vi "field emission sensor_v72.vi"() -> ()   [LabVIEW 2014]
uses:
  Keithley 24XX/Public/Data/Read (Single Point).vi
  Keithley 24XX/Keithley 24XX.lvlib
  <userlib>/Nanonis Prog Interface V5/Nanonis Prog Interface.lvlib
  <vilib>/Analysis/NI_AALBase.lvlib
panel:
  in  "p Current Amplitude (A)":dbl=-0.3 format="%#_6p"
  in  "Current Amplitude Max (A)":sgl=1.5e-10 format="%#_6p"
  in  "Std threshold":dbl=5e-12 format="%#_6p"
  in  "Mean threshold":dbl=2e-11 format="%#_6p"
  out "ramp paused":bool
  out "x+y":sgl=1.4799449e-10
  out "amplitude":sgl(graph)=1.0739469e-11
  in  "Amplitude (V) (NaN=no change)":sgl=nan
  in  "Frequency (Hz) (NaN=no change)":sgl=nan format="%#_6p"
  in  "p Amplitude":dbl=-0.3 format="%#_6p"
  in  "amplitude max":sgl=1.5e-10 format="%#_6p"
  in  "Signal index (0-79)":i8=49
  out "amplitude":sgl=1.0739469e-11 format="%#_6p"
  in  "dz":dbl=1e-09 format="%#_6p"
  in  "ramp delay (s)":dbl=0.001
  out "ramp trigger":bool
  out "millisecond timer value":u32=272952714
  in  "Clear plots":bool
  out "z":dbl(graph)=7.783200430924225e-08
  in  "Ramp":bool
  in  "steps":sgl=5e-09 format="%#_6p"
  in  "Ramp to":sgl=1.3e-06 format="%#_6p"
  in  "I":sgl=5e-05 format="%#_6p"
  in  "PID":bool
  in  "p":sgl=0.01 format="%#_6p"
  in  "setpoint":sgl format="%#_3p"
  in  "max Current":sgl=2e-06 format="%#_6p"
  in  "setpoint approach":sgl=3e-08 format="%#_6p"
  in  "auto approach":bool
  in  "Number of steps":u16=1
  in  "withdraw tip":bool
  in  "coarse step":bool
  in  "Direction":enum16{"X +", "X -", "Y +", "Y -", "Z +", "Z -"}(ring)=enum."Z +"
  in  "Machine name (local machine IP)":string="localhost"
  in  "Z position [m]":dbl=7.783200430924225e-08 max=1.096e-07 step=1.0 format="%_6p"
  out "current [A]":sgl=-1.479945e-08 format="%#_6p"
  in  "time divider":dbl=60.0
  out "time elapsed":dbl=72.48559594154358
  in  "milliseconds to wait":u32=100
  in  "VISA resource name":refnum<visa-resource-name>="GPIB0::21::INSTR"
  in  "stop":bool
  in  "current multiplier":sgl=1.0
  out "Current":sgl(graph)=-1.479945e-08
  # "STOP the VI during an Nanonis Auto Approach"
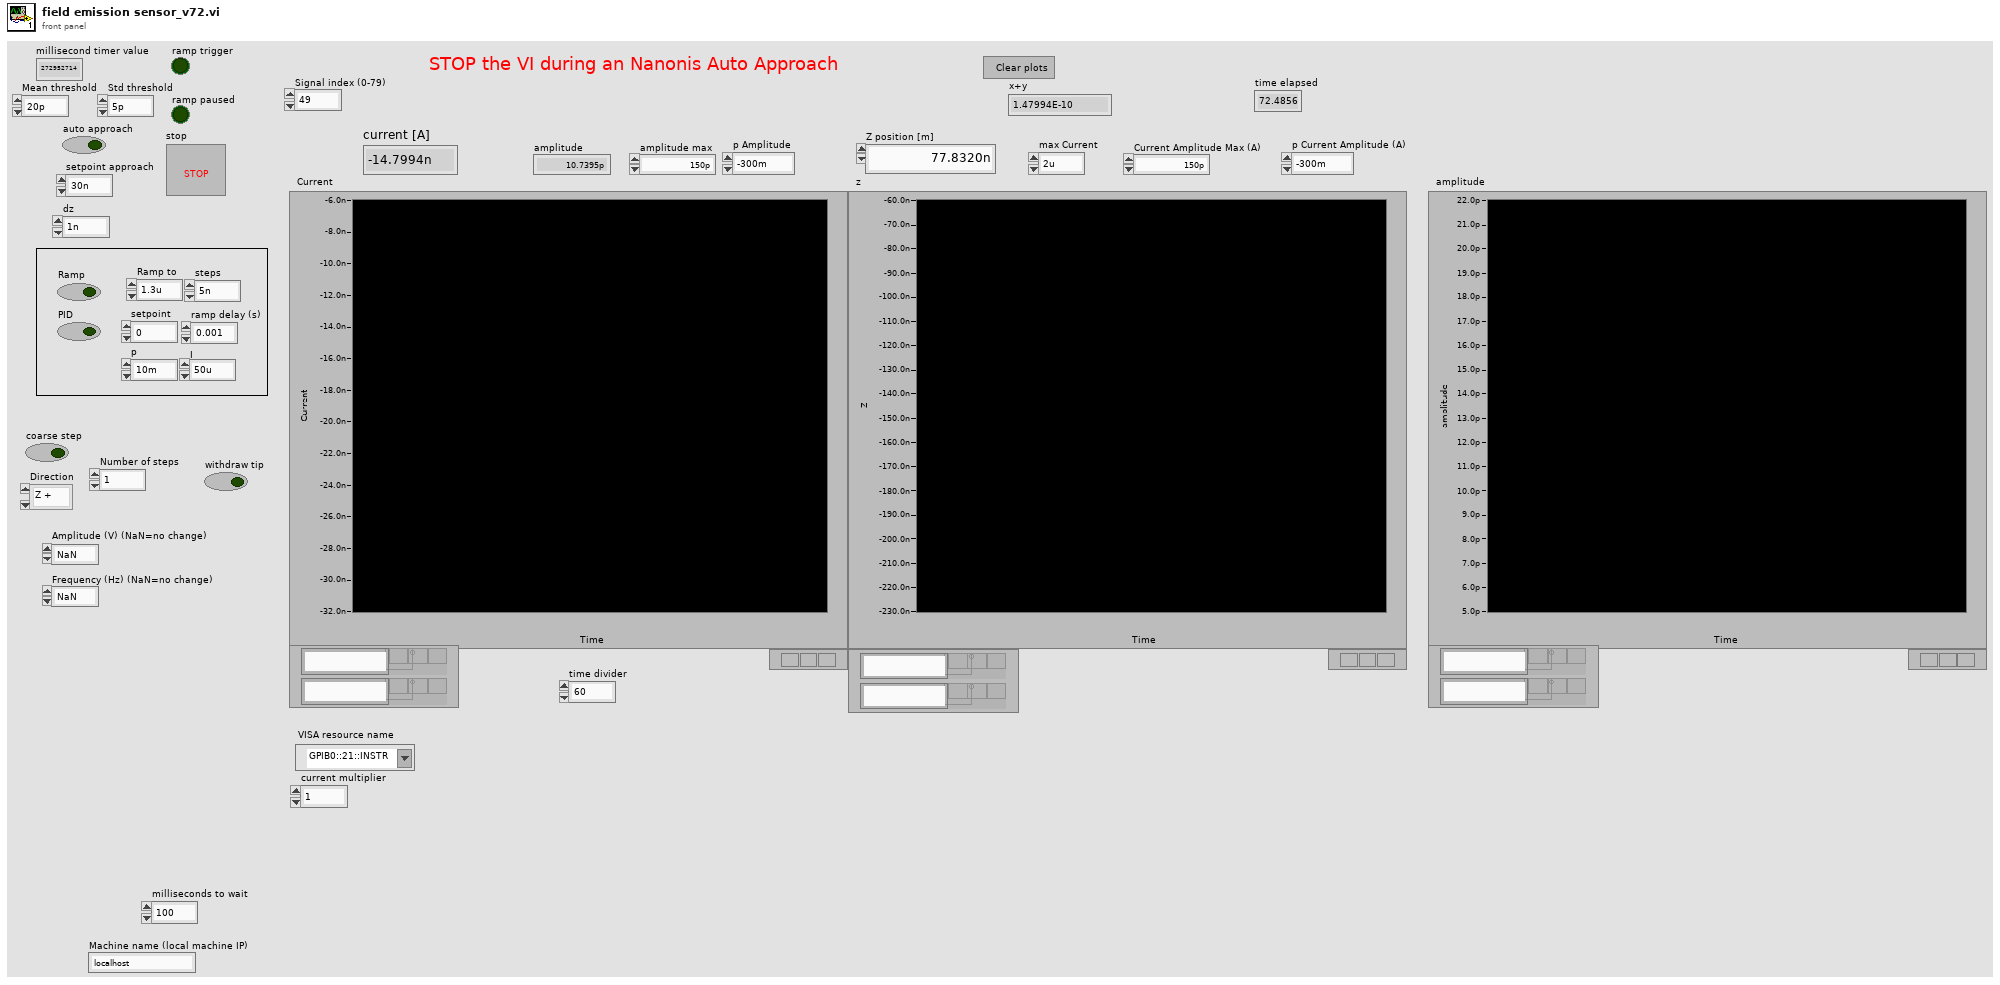
[diagram p1: front panel]
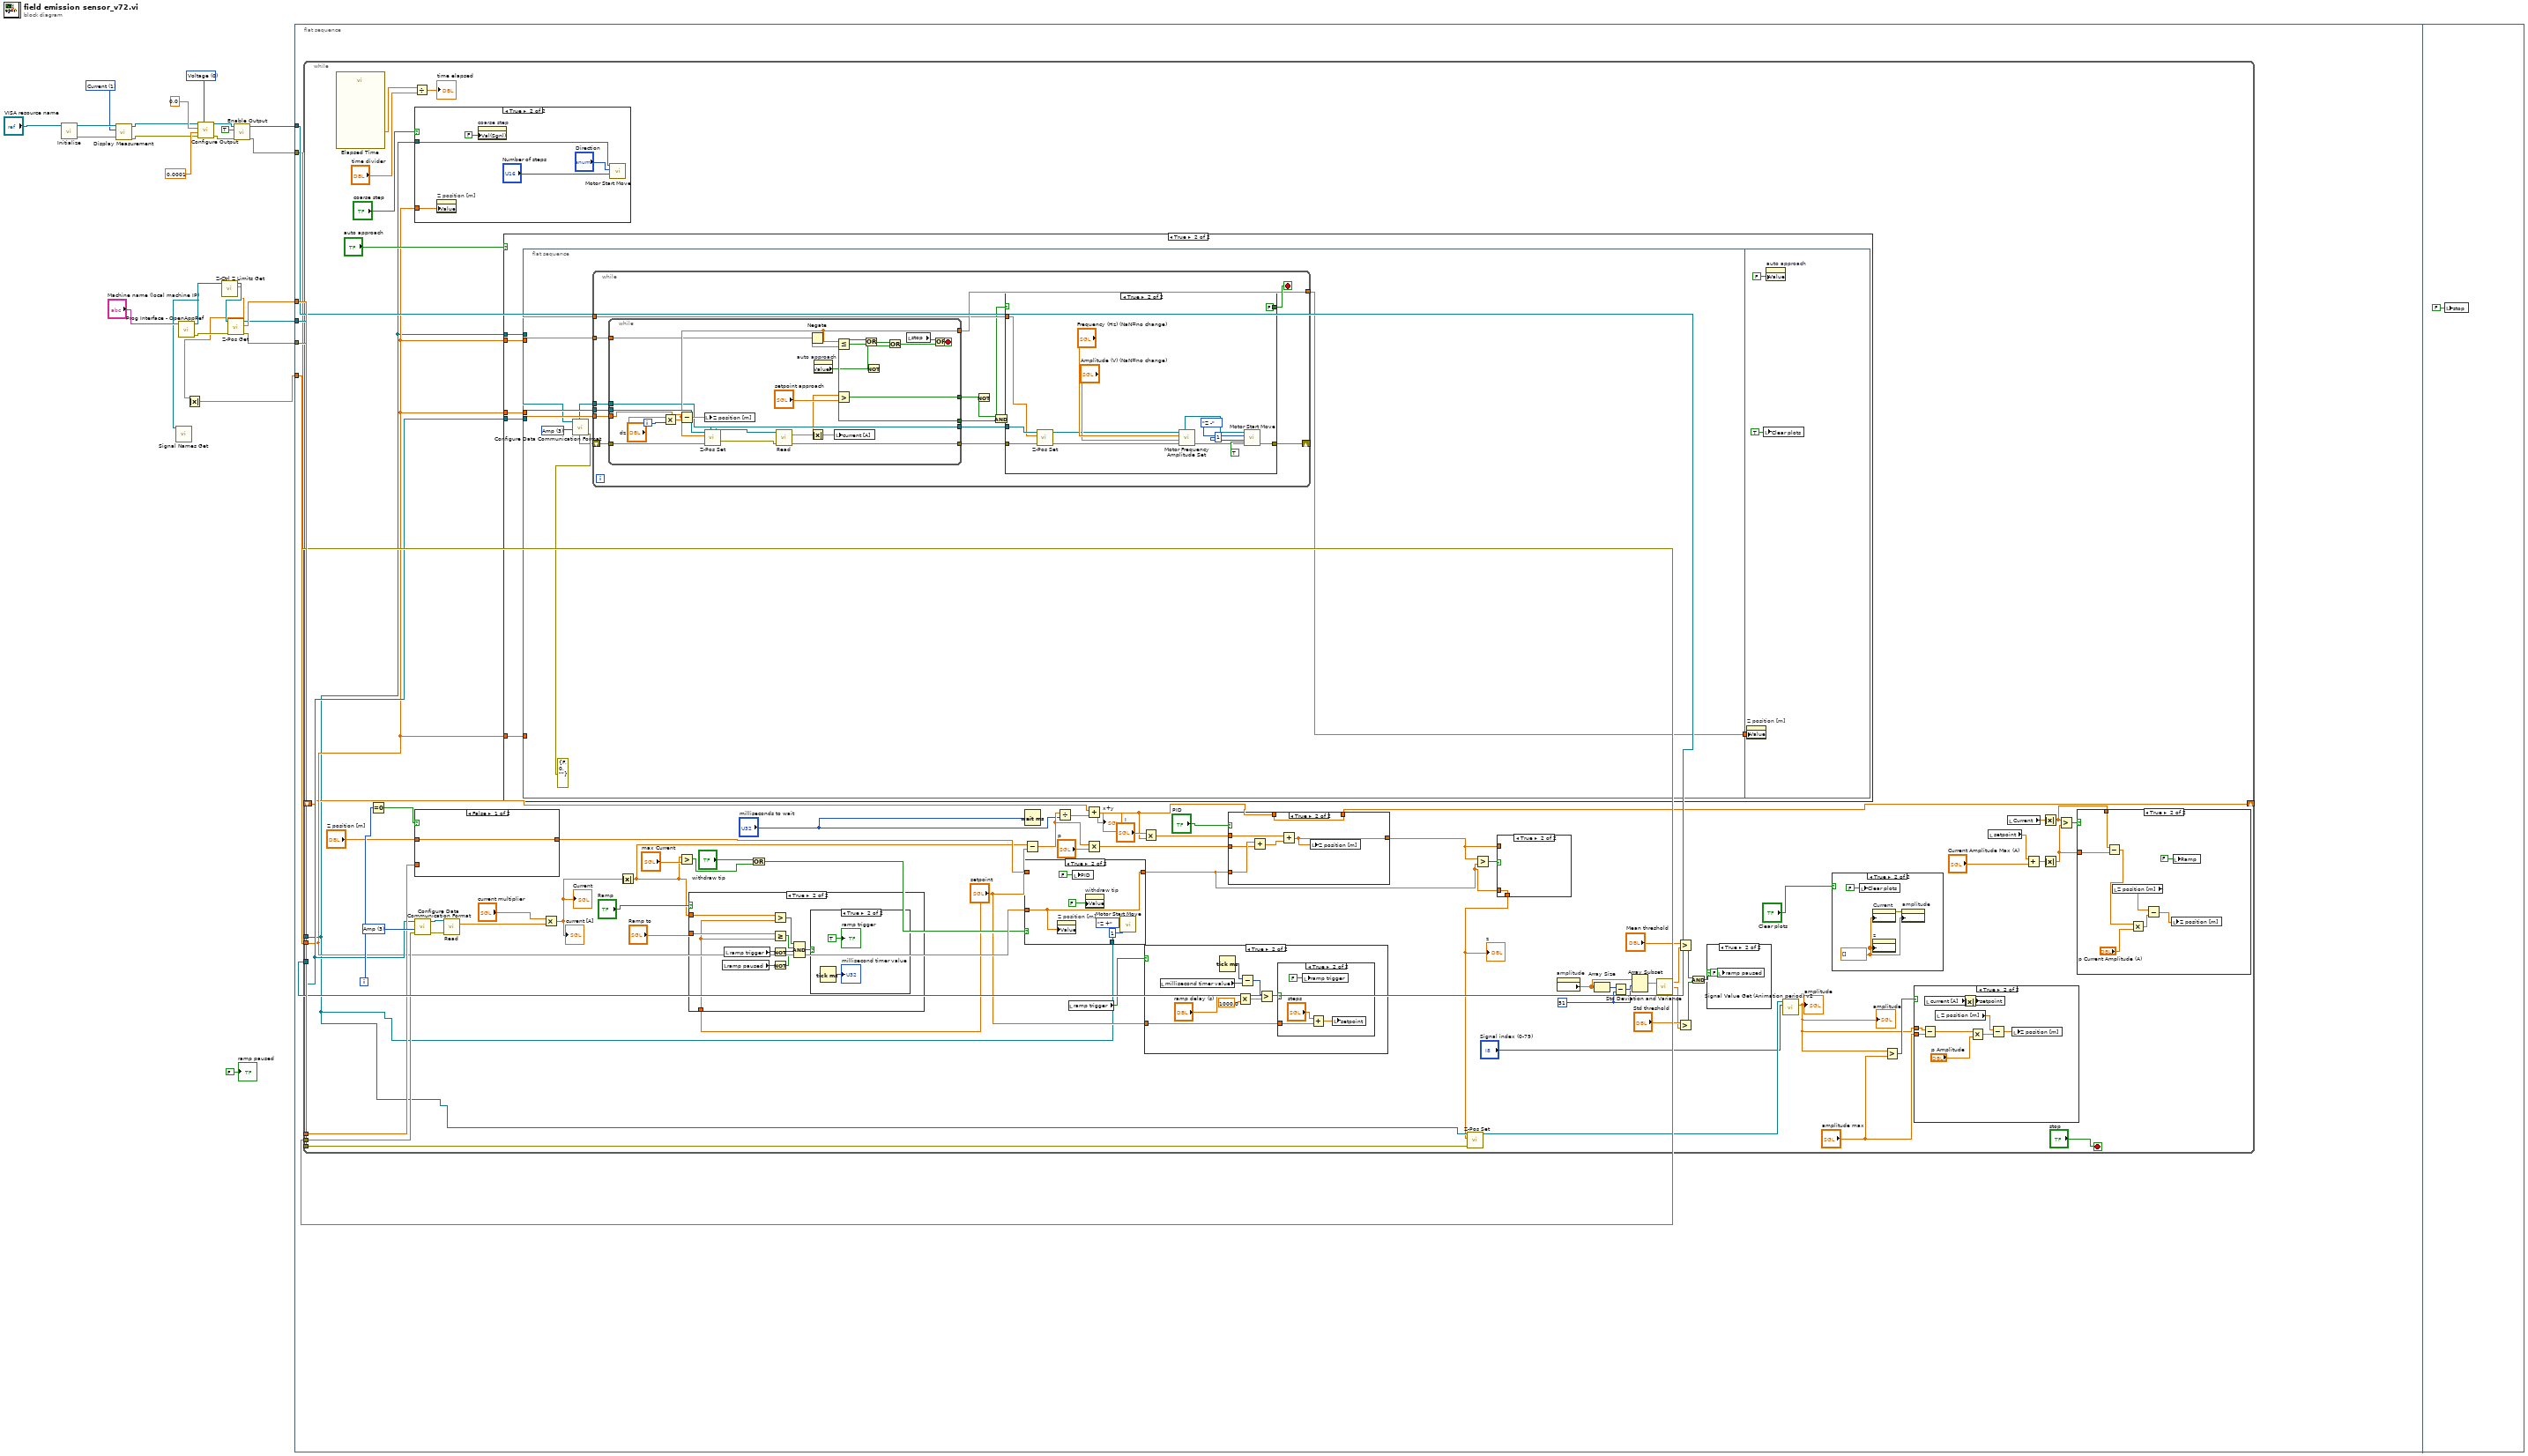
[diagram p0: block diagram]
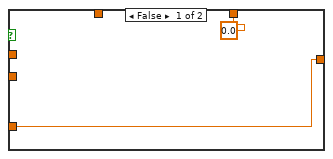
[diagram p11: hidden frame]
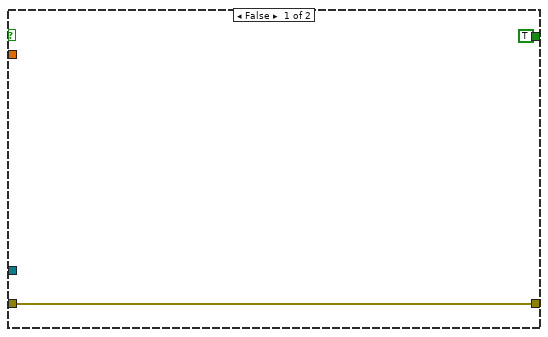
[diagram p13: hidden frame]
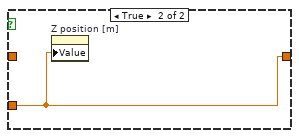
[diagram p16: hidden frame]
diagram:
  w6 = u16 1 items=["Voltage", "Current", "Resistance"] ("Displayed Measurement (0: Voltage)")
  w18 = u16 0 items=["Voltage", "Current"] ("Source Mode  (0: Voltage)")
  n1 = call "Initialize.vi"("VISA resource name"="VISA resource name") -> ("error out"=w8:errorcluster, "VISA resource name out"=w10:refnum<visa-resource-name>)  [unwired: 9 in]
  n2 = call "Display Measurement.vi"("error in (no error)"=w8, "Displayed Measurement (0: Voltage)"=w6, "VISA resource name"=w10) -> ("error out"=w7:errorcluster, "VISA resource name out"=w9:refnum<visa-resource-name>)  [unwired: 7 in]
  n3 = call <userlib>:"Prog Interface - OpenAppRef.vi"("Machine name (local machine IP)"="Machine name (local machine IP)") -> ("Error out"=w23:errorcluster, "Application reference"=w2:refnum<vi>)  [unwired: 5 in]
  n4 = call <userlib>:"Signal Names Get.vi"("Application ref in"=w2) -> ()  [unwired: 6 in, 3 out]
  n5 = call "Configure Output.vi"("Source Mode  (0: Voltage)"=w18, "error in (no error)"=w7, "Compliance  Level (0.1)"=0.0001, "Output Level (0)"=0.0, "VISA resource name"=w9) -> ("error out"=w14:errorcluster, "VISA resource name out"=w15:refnum<visa-resource-name>)  [unwired: 5 in]
  n6 = call <userlib>:"Z-Ctrl Z Limits Get.vi"("Application ref in"=w2) -> ("Z high limit"=w3:sgl, "Application ref out"=w4:refnum<vi>)  [unwired: 7 in, 2 out]
  n7 = Absolute Value(x=w3) -> (abs(x)=w5:sgl)
  n8 = call <userlib>:"Z-Pos Get.vi"("error in (no error)"=w23, "Application ref in"=w4) -> ("error out"=w22:errorcluster, "Z position (m)"=w21:sgl, "Application ref out"=w20:refnum<vi>)  [unwired: 7 in]
  n9 = call "Enable Output.vi"("error in (no error)"=w14, "Enable Output (T: Enable)"=TRUE, "VISA resource name"=w15) -> ("error out"=w11:errorcluster, "VISA resource name out"=w12:refnum<visa-resource-name>)  [unwired: 7 in]
  n10 = flat-sequence {
    tunnel: w22 -> [w30]
    tunnel: w21 -> [w29]
    tunnel: w20 -> [w28]
    tunnel: w12 -> [w27]
    tunnel: w11 -> [w26]
    tunnel: w5 -> [w25]
    frame #0 {
      n11 = while {
        tunnel: w28 -> [w54]
        tunnel: w30 -> [w93]
        tunnel: w29 -> [w92]
        tunnel: w27 -> [w84]
        tunnel: w26 -> [w83]
        tunnel: w25 -> [w81]
        shift-right: [w66] -> _
        shift-left: _ -> [w73]
        i -> [w91]
        stop <- "stop" stop-if-true
        w46 = 51 ("y")
        w97 = u16 3 items=["All", "Volt and Amp", "Volt", "Amp"] ("Data Selection (0: All)")
        n12 = call "Elapsed Time"() -> ("Elapsed Time (s)"=w94:dbl)  [unwired: 12 in, 7 out]
        n13 = Equal To 0?(x=w91) -> (x = 0?=w90:bool)
        n14 = Divide(x=w94, y="time divider") -> (x/y=→"time elapsed":dbl)
        n15 = case shown="True" "coarse step" {
          tunnel: w54 -> [_ w242]
          tunnel: w81 -> [_ w238]
          frame False {
          }
          frame True {
            n16 = property on="Z position [m]" class="DigNum (strict)"("Value"=w238) -> ()  [unwired: 2 in, 2 out]
            n17 = property on="coarse step" class="Bool (strict)"("Val(Sgnl)"=FALSE ("Value (Signaling)")) -> ()  [unwired: 2 in, 2 out]
            n18 = call <userlib>:"Motor Start Move.vi"("Number of steps"="Number of steps", "Direction"="Direction", "Application ref in"=w242) -> ()  [unwired: 6 in, 2 out]
          }
        }
        n19 = case shown="False" w90 {
          tunnel: [w243 w244] -> w87
          tunnel: w92 -> [_ w244]
          tunnel: "Z position [m]" -> [w243 _]
          frame False {
          }
          frame True {
            n20 = property on="Z position [m]" class="DigNum (strict)"("Value"=w244) -> ()  [unwired: 2 in, 2 out]
          }
        }
        n21 = call "Configure Data Communication Format.vi"("error in (no error)"=w83, "Data Selection (0: All)"=w97, "VISA resource name"=w84) -> ("error out"=w98:errorcluster, "VISA resource name out"=w99:refnum<visa-resource-name>)  [unwired: 7 in]
        n22 = call-poly "Read.vi"("VISA resource name"=w99, "error in (no error)"=w98) -> ("Current"=w101:sgl)  [unwired: 7 in, 6 out]
        n23 = case shown="True" "auto approach" {
          tunnel: w84 -> [_ w162]
          tunnel: w54 -> [_ w161]
          tunnel: w81 -> [_ w159]
          tunnel: w81 -> [_ w158]
          tunnel: w81 -> [_ w157]
          frame False {
          }
          frame True {
            n24 = flat-sequence {
              tunnel: w162 -> [w165]
              tunnel: w161 -> [w172]
              tunnel: [w171] -> w160
              tunnel: w159 -> [w170]
              tunnel: w158 -> [w169]
              tunnel: w157 -> [w168]
              tunnel: w160 -> [w229]
              frame #0 {
                w163 = u16 3 items=["All", "Volt and Amp", "Volt", "Amp"] ("Data Selection (0: All)")
                n25 = call "Configure Data Communication Format.vi"("error in (no error)"=errorcluster {"status"=FALSE, "code"=0, "source"=""}, "Data Selection (0: All)"=w163, "VISA resource name"=w165) -> ("error out"=w166:errorcluster, "VISA resource name out"=w164:refnum<visa-resource-name>)  [unwired: 7 in]
                n26 = while {
                  tunnel: w164 -> [w187]
                  tunnel: w172 -> [w186]
                  tunnel: [w180] -> w171
                  tunnel: w170 -> [w179]
                  tunnel: w169 -> [w178]
                  tunnel: w168 -> [w177]
                  shift-right: [w176] -> _
                  shift-left: w166 -> [w175]
                  stop <- w181 stop-if-true
                  n27 = while {
                    tunnel: w187 -> [w205]
                    tunnel: w186 -> [w225]
                    tunnel: [w224] -> w185
                    tunnel: [w223] -> w184
                    tunnel: [w222] -> w183
                    tunnel: [w207] -> w182
                    tunnel: [w221] -> w180
                    tunnel: w179 -> [w220]
                    tunnel: w177 -> [w218]
                    tunnel: w175 -> [w206]
                    i -> [w227]
                    stop <- w213 stop-if-true
                    n28 = Multiply(x="dz", y=w227) -> (x*y=w209:dbl)
                    n29 = Subtract(x=w220, y=w209) -> (x-y=w221:dbl)
                    n30 = local write "Z position [m]"(w221) -> ()
                    n31 = call <userlib>:"Z-Pos Set.vi"("error in (no error)"=w206, "Z position (m)"=w221, "Application ref in"=w225) -> ("error out"=w204:errorcluster, "Application ref out"=w222:refnum<vi>)  [unwired: 7 in]
                    n32 = call-poly "Read.vi"("VISA resource name"=w205, "error in (no error)"=w204) -> ("Current"=w226:sgl, "error out"=w207:errorcluster)  [unwired: 7 in, 5 out]
                    n33 = Negate(x=w218) -> (-x=w219:sgl)
                    n34 = Absolute Value(x=w226) -> (abs(x)=w210:sgl)
                    n35 = property on="auto approach" class="Bool (strict)"() -> ("Value"=w216:bool)  [unwired: 2 in, 2 out]
                    n36 = local write "current [A]"(w210) -> ()
                    n37 = Less Or Equal?(x=w221, y=w219) -> (x <= y?=w223:bool)
                    n38 = Greater?(x=w210, y="setpoint approach") -> (0:w224:bool)
                    n39 = Or(x=w224, y=w223) -> (x .or. y?=w217:bool)
                    n40 = Not(x=w216) -> (.not. x?=w215:bool)
                    n41 = Or(x=w217, y=w215) -> (x .or. y?=w214:bool)
                    n42 = local read "stop"() -> (w212:bool)
                    n43 = Or(x=w212, y=w214) -> (x .or. y?=w213:bool)
                  }
                  n44 = Not(x=w185) -> (.not. x?=w174:bool)
                  n45 = And(x=w174, y=w184) -> (x .and. y?=w173:bool)
                  n46 = case shown="True" w173 {
                    tunnel: w183 -> [_ w203]
                    tunnel: w182 -> [w188 w202]
                    tunnel: [TRUE FALSE] -> w181
                    tunnel: w178 -> [_ w198]
                    tunnel: [w188 w191] -> w176
                    frame False {
                    }
                    frame True {
                      n47 = call <userlib>:"Z-Pos Set.vi"("error in (no error)"=w202, "Z position (m)"=w198, "Application ref in"=w203) -> ("error out"=w195:errorcluster, "Application ref out"=w190:refnum<vi>)  [unwired: 7 in]
                      n48 = call <userlib>:"Motor Frequency Amplitude Set.vi"("Error in (no error)"=w195, "Amplitude (V) (NaN=no change)"="Amplitude (V) (NaN=no change)", "Frequency (Hz) (NaN=no change)"="Frequency (Hz) (NaN=no change)", "Application ref in"=w190) -> ("Error out"=w194:errorcluster, "Application ref out"=w196:refnum<vi>)  [unwired: 6 in]
                      n49 = call <userlib>:"Motor Start Move.vi"("Wait until finished? (F)"=TRUE, "Error in (no error)"=w194, "Number of steps"=u16 1, "Direction"=enum16{"X +", "X -", "Y +", "Y -", "Z +", "Z -"}."Z -", "Application ref in"=w196) -> ("Error out"=w191:errorcluster)  [unwired: 4 in, 1 out]
                    }
                  }
                }
              }
              frame #1 {
                n50 = property on="Z position [m]" class="DigNum (strict)"("Value"=w229) -> ()  [unwired: 2 in, 2 out]
                n51 = local write "Clear plots"(TRUE ("Clear plots")) -> ()
                n52 = property on="auto approach" class="Bool (strict)"("Value"=FALSE ("auto approach")) -> ()  [unwired: 2 in, 2 out]
              }
            }
          }
        }
        n53 = Multiply(x="current multiplier", y=w101) -> (x*y=w80:sgl)
        "Current" <- w80
        "current [A]" <- w80
        n54 = Absolute Value(x=w80) -> (abs(x)=w64:sgl)
        n55 = Greater?(x=w64, y="max Current") -> (0:w77:bool)
        n56 = case shown="True" "Ramp" {
          tunnel: w64 -> [_ w146]
          tunnel: "setpoint" -> [_ w143]
          tunnel: "Ramp to" -> [_ w144]
          frame False {
          }
          frame True {
            n57 = local read "ramp paused"() -> (w138:bool)
            n58 = local read "ramp trigger"() -> (w140:bool)
            n59 = Greater?(x=w146, y=w143) -> (0:w145:bool)
            n60 = Greater Or Equal?(x=w144, y=w143) -> (x >= y?=w141:bool)
            n61 = Not(x=w140) -> (.not. x?=w139:bool)
            n62 = Not(x=w138) -> (.not. x?=w137:bool)
            n63 = Compound Arithmetic op=AND(w145, w141, w139, w137) -> (w142:bool)
            n64 = case shown="True" w142 {
              frame False {
              }
              frame True {
                n65 = Tick Count (ms)() -> (millisecond timer value=→"millisecond timer value":u32)
                "ramp trigger" <- TRUE ("ramp")
              }
            }
          }
        }
        n66 = Or(x="withdraw tip", y=w77) -> (x .or. y?=w78:bool)
        n67 = Subtract(x=w64, y="setpoint") -> (x-y=w69:sgl)
        n68 = Wait (ms)(milliseconds to wait="milliseconds to wait") -> ()  [unwired: 1 out]
        n69 = case shown="True" w78 {
          tunnel: [w231 w236] -> w50
          tunnel: w87 -> [w231 _]
          tunnel: w81 -> [_ w236]
          tunnel: w54 -> [_ w234]
          frame False {
          }
          frame True {
            n70 = property on="Z position [m]" class="DigNum (strict)"("Value"=w236) -> ()  [unwired: 2 in, 2 out]
            n71 = local write "PID"(FALSE ("PID")) -> ()
            n72 = property on="withdraw tip" class="Bool (strict)"("Value"=FALSE ("withdraw tip")) -> ()  [unwired: 2 in, 2 out]
            n73 = call <userlib>:"Motor Start Move.vi"("Number of steps"=u16 1, "Direction"=enum16{"X +", "X -", "Y +", "Y -", "Z +", "Z -"}."Z +", "Application ref in"=w234) -> ()  [unwired: 6 in, 2 out]
          }
        }
        n74 = Divide(x=w69, y="milliseconds to wait") -> (x/y=w70:sgl)
        n75 = local read "ramp trigger"() -> (w60:bool)
        n76 = Add(x=w73, y=w70) -> (x+y=w67:sgl)
        "x+y" <- w67
        n77 = Multiply(x=w69, y="p") -> (x*y=w74:sgl)
        n78 = Multiply(x="I", y=w67) -> (x*y=w71:sgl)
        n79 = case shown="True" w60 {
          tunnel: "setpoint" -> [_ w125]
          frame False {
          }
          frame True {
            n80 = local read "millisecond timer value"() -> (w128:u32)
            n81 = Tick Count (ms)() -> (millisecond timer value=w129:u32)
            n82 = Multiply(x="ramp delay (s)", y=1000.0) -> (x*y=w122:dbl)
            n83 = Subtract(x=w129, y=w128) -> (x-y=w127:u32)
            n84 = Greater?(x=w127, y=w122) -> (0:w126:bool)
            n85 = case shown="True" w126 {
              tunnel: w125 -> [_ w131]
              frame False {
              }
              frame True {
                n86 = local write "ramp trigger"(FALSE ("ramp")) -> ()
                n87 = Add(x="steps", y=w131) -> (x+y=w133:sgl)
                n88 = local write "setpoint"(w133) -> ()
              }
            }
          }
        }
        n89 = case shown="True" "PID" {
          tunnel: w50 -> [w150 w156]
          tunnel: [w150 w152] -> w52
          tunnel: w74 -> [_ w155]
          tunnel: w71 -> [_ w153]
          tunnel: w67 -> [_ w151]
          tunnel: [sgl 0.0 w151] -> w66
          frame False {
          }
          frame True {
            n90 = Add(x=w156, y=w155) -> (x+y=w154:dbl)
            n91 = Add(x=w153, y=w154) -> (x+y=w152:dbl)
            n92 = local write "Z position [m]"(w152) -> ()
          }
        }
        n93 = Greater?(x=w52, y=w50) -> (0:w53:bool)
        n94 = case shown="True" w53 {
          tunnel: w52 -> [w111 _]
          tunnel: [w111 w112] -> w51
          tunnel: w50 -> [_ w112]
          frame False {
          }
          frame True {
          }
        }
        "z" <- w51
        n95 = call <userlib>:"Z-Pos Set.vi"("error in (no error)"=w93, "Z position (m)"=w51, "Application ref in"=w54) -> ("Application ref out"=w59:refnum<vi>)  [unwired: 7 in, 1 out]
        n96 = property on="amplitude" class="WFChart (strict)"() -> ("History Data"=w49:sgl[])  [unwired: 2 in, 2 out]
        n97 = Array Size(array=w49) -> (size(s)=w48:i32)
        n98 = Subtract(x=w48, y=w46) -> (x-y=w47:i32)
        n99 = Array Subset(array=w49, index=w47, length=w46) -> (w45:sgl[])
        n100 = call <vilib>:"Std Deviation and Variance.vi"("X"=w45) -> ("mean"=w44:dbl, "standard deviation"=w38:dbl)  [unwired: 1 in, 1 out]
        n101 = Greater?(x="Mean threshold", y=w44) -> (0:w40:bool)
        n102 = Greater?(x="Std threshold", y=w38) -> (0:w41:bool)
        n103 = And(x=w40, y=w41) -> (x .and. y?=w39:bool)
        n104 = case shown="True" w39 {
          frame False {
          }
          frame True {
            n105 = local write "ramp paused"(FALSE ("ramp paused")) -> ()
          }
        }
        n106 = call <userlib>:"Signal Value Get (Animation period) v2.vi"("Signal index (0-79)"="Signal index (0-79)", "Application ref in"=w59) -> ("Signal value"=w56:sgl)  [unwired: 6 in, 2 out]
        "amplitude" <- w56
        "amplitude" <- w56
        n107 = case shown="True" "Clear plots" {
          frame False {
          }
          frame True {
            w134 = dbl[] [] ("History Data")
            n108 = local write "Clear plots"(FALSE ("Clear plots")) -> ()
            n109 = property on="Current" class="WFChart (strict)"("History Data"=w134) -> (error out=w135:errorcluster)  [unwired: 2 in, 1 out]
            n110 = property on="z" class="WFChart (strict)"("History Data"=w134) -> ()  [unwired: 2 in, 2 out]
            n111 = property on="amplitude" class="WFChart (strict)"(error in=w135, "History Data"=w134) -> ()  [unwired: 1 in, 2 out]
          }
        }
        n112 = Greater?(x=w56, y="amplitude max") -> (0:w57:bool)
        n113 = case shown="True" w57 {
          tunnel: w56 -> [_ w119]
          tunnel: "amplitude max" -> [_ w118]
          frame False {
          }
          frame True {
            n114 = Subtract(x=w119, y=w118) -> (x-y=w117:sgl)
            n115 = local read "current [A]"() -> (w114:sgl)
            n116 = local read "Z position [m]"() -> (w121:dbl)
            n117 = Absolute Value(x=w114) -> (abs(x)=w113:sgl)
            n118 = Multiply(x=w117, y="p Amplitude") -> (x*y=w115:dbl)
            n119 = local write "setpoint"(w113) -> ()
            n120 = Subtract(x=w121, y=w115) -> (x-y=w120:dbl)
            n121 = local write "Z position [m]"(w120) -> ()
          }
        }
        n122 = local read "setpoint"() -> (w34:sgl)
        n123 = local read "Current"() -> (w33:sgl)
        n124 = Add(x=w34, y="Current Amplitude Max (A)") -> (x+y=w36:sgl)
        n125 = Absolute Value(x=w33) -> (abs(x)=w32:sgl)
        n126 = Absolute Value(x=w36) -> (abs(x)=w31:sgl)
        n127 = Greater?(x=w32, y=w31) -> (0:w35:bool)
        n128 = case shown="True" w35 {
          tunnel: w32 -> [_ w108]
          tunnel: w31 -> [_ w106]
          frame False {
          }
          frame True {
            n129 = Subtract(x=w108, y=w106) -> (x-y=w107:sgl)
            n130 = local read "Z position [m]"() -> (w104:dbl)
            n131 = Multiply(x=w107, y="p Current Amplitude (A)") -> (x*y=w105:dbl)
            n132 = Subtract(x=w104, y=w105) -> (x-y=w103:dbl)
            n133 = local write "Z position [m]"(w103) -> ()
            n134 = local write "Ramp"(FALSE ("Ramp")) -> ()
          }
        }
      }
    }
    frame #1 {
      n135 = local write "stop"(FALSE ("stop")) -> ()
    }
  }
  "ramp paused" <- FALSE ("ramp paused")
